vi "Matches.vi"(8 "error in (no error)":errorcluster, 10 "Actual":variant, 11 "Count in":refnum<class "Count.lvclass">) -> (0 "error out":errorcluster, 2 "Result":bool, 3 "Count out":refnum<class "Count.lvclass">)   [LabVIEW 2017, in "Transparent Assertions.lvlib" / "Constraints.lvlib" / "Count.lvclass"]
doc: "Evaluates the constraint for <B>Actual</B>. Returns true if the constraint is met."
uses:
  Count.lvclass
  Count.lvclass/Count.ctl
  Constraints.lvlib
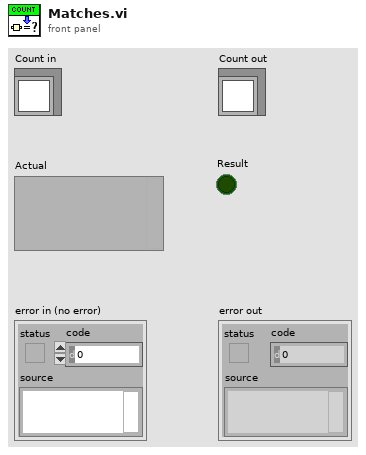
[diagram p1: front panel]
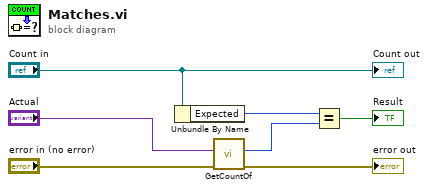
[diagram p0: block diagram]
diagram:
  n1 = Unbundle By Name("Count in") -> ("Expected"=w1:i32)
  n2 = call "GetCountOf.vi"("error in (no error)"="error in (no error)", "Countable"="Actual") -> ("error out"=→"error out":errorcluster, "Count"=w4:i32)  [unwired: 8 in]
  n3 = Equal?(x=w1, y=w4) -> (x = y?=→"Result":bool)
  "Count out" <- "Count in"
